vi "get Font Pointer.vi"(8 "error in (no error)":errorcluster, 10 "Font Combo":string, 11 "Resource Manager in":refnum<class "Resource Manager.lvclass">) -> (0 "error out":errorcluster, 2 "Font Pointer":u32 format="%.0x", 3 "Resource Manager out":refnum<class "Resource Manager.lvclass">)   [LabVIEW 2015, in "Resource Manager.lvclass"]
uses:
  Resource Manager.lvclass
  Resource Manager.lvclass/Resource Manager.ctl
  LabSDL2/Source/Libraries/LibSDL2_TTF Wrapper/LibSDL2_TTF.lvlib
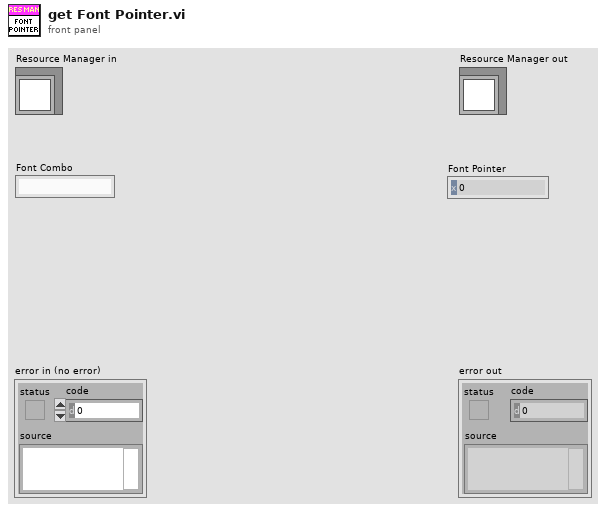
[diagram p1: front panel]
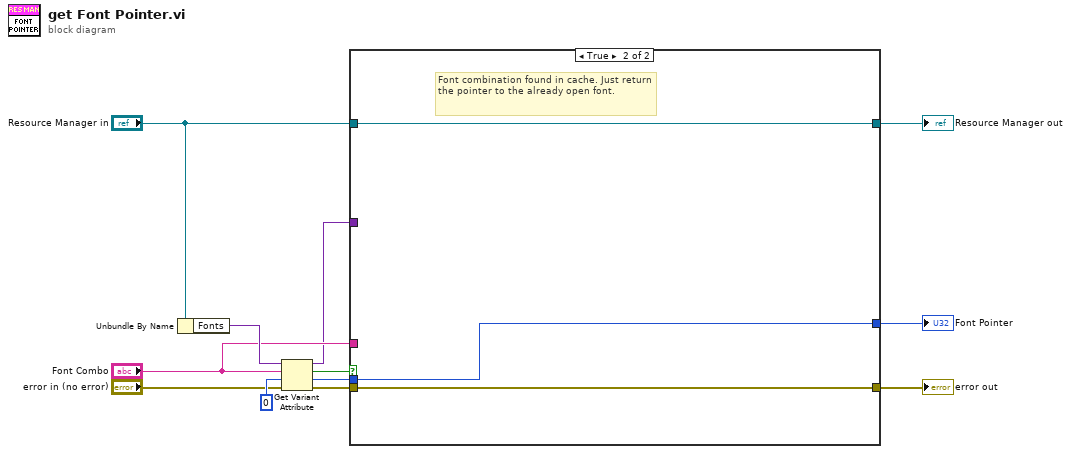
[diagram p0: block diagram]
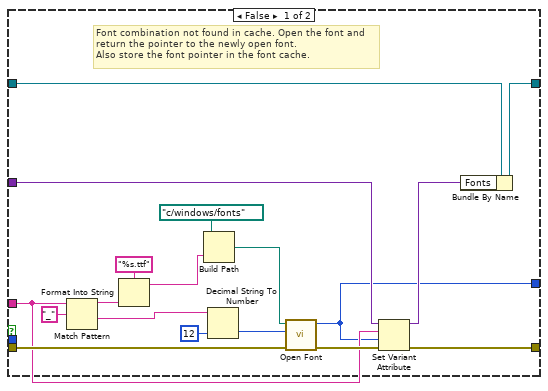
[diagram p2: hidden frame]
diagram:
  n1 = Unbundle By Name("Resource Manager in") -> ("Fonts"=w11:variant)
  n2 = Get Variant Attribute(Variant=w11, name="Font Combo", default value (empty Variant)=u32 0 ("Font Pointer"), error in="error in (no error)") -> (duplicate Variant=w1:variant, found=w9:bool, value=w4:u32, error out=w6:errorcluster)
  n3 = case shown="True" w9 {
    tunnel: [w16 w33] -> w8
    tunnel: "Resource Manager in" -> [w17 w33]
    tunnel: w6 -> [w30 w32]
    tunnel: [w19 w32] -> w5
    tunnel: w4 -> [_ w31]
    tunnel: [w13 w31] -> w3
    tunnel: "Font Combo" -> [w14 _]
    tunnel: w1 -> [w18 _]
    frame False {
      # "Font combination not found in cache. Open the font and return the pointer to the newly open font.\nAlso store the font pointer in the font cache."
      n4 = Match Pattern(string=w14, regular expression="_") -> (before substring=w25:string, after substring=w23:string)  [unwired: 1 in, 2 out]
      n5 = Format Into String(format string="%s.ttf", w25) -> (resulting string=w24:string)  [unwired: 2 in, 1 out]
      n6 = Build Path(base path=path "c:/windows/fonts" ("File"), name or relative path=w24) -> (appended path=w29:path)
      n7 = Decimal String To Number(string=w23, default (0L)=12 ("default (0 I32)")) -> (number=w21:i32)  [unwired: 1 in, 1 out]
      n8 = call "Open Font.vi"("error in (no error)"=w30, "Size"=w21, "File"=w29) -> ("error out"=w20:errorcluster, "Font Pointer"=w13:u32)  [unwired: 7 in]
      n9 = Set Variant Attribute(Variant=w18, name=w14, value=w13, error in=w20) -> (Variant out=w15:variant, error out=w19:errorcluster)  [unwired: 1 out]
      n10 = Bundle By Name(cluster=w17, "Fonts"=w15) -> (w16:refnum<class "Resource Manager.lvclass">)
    }
    frame True {
      # "Font combination found in cache. Just return the pointer to the already open font."
    }
  }
  "error out" <- w5
  "Resource Manager out" <- w8
  "Font Pointer" <- w3
